vi "Get Ref Prop.vi"(8 "error in (no error)":errorcluster, 11 "VariableContainer in":refnum<class "VariableContainer.lvclass">) -> (0 "error out":errorcluster, 2 "Ref":refnum<k7>, 3 "VariableContainer out":refnum<class "VariableContainer.lvclass">)   [LabVIEW 2020, in "TSS.lvlib" / "VariableContainer.lvclass"]
uses:
  VariableContainer.lvclass
  VariableContainer.lvclass/VariableContainer.ctl
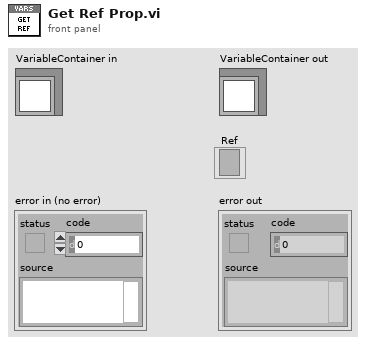
[diagram p1: front panel]
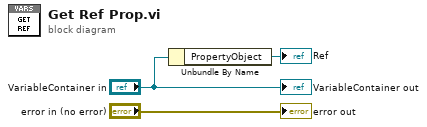
[diagram p0: block diagram]
diagram:
  n1 = Unbundle By Name("VariableContainer in") -> ("PropertyObject"=→"Ref":refnum<k7>)
  "error out" <- "error in (no error)"
  "VariableContainer out" <- "VariableContainer in"
